vi "ql2_id_to_query.vi"(11 "id":u32) -> (3 "query_type":T1)   [LabVIEW 2017, in "rethinkdb.lvlib"]
uses:
  ql2_query.ctl
  rethinkdb.lvlib
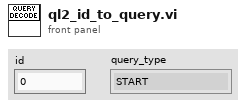
[diagram p1: front panel]
types:
  T1 = typedef "rethinkdb.lvlib/ql2_query.ctl" = enum8{"START", "CONTINUE", "STOP", "NOREPLY_WAIT", "SERVER_INFO", "invalid"}
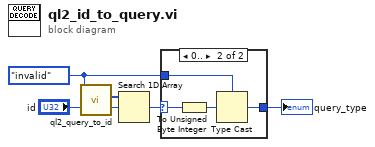
[diagram p0: block diagram]
diagram:
  w1 = ql2_query."invalid" ("query_type")
  n1 = call "ql2_query_to_id.vi"("query_type"=w1) -> ("query_type_ids"=w2:u32[])  [unwired: 9 in, 1 out]
  n2 = Search 1D Array(1D array=w2, element="id") -> (index of element=w4:i32)  [unwired: 1 in]
  n3 = case shown="0.." w4 {
    selector: w4 -> [_ w7]
    tunnel: [w6 w10] -> w3
    tunnel: w1 -> [w6 w9]
    frame ..-1 {
    }
    frame 0.. {
      n4 = To Unsigned Byte Integer(number=w7) -> (unsigned 8bit integer=w8:u8)
      n5 = Type Cast(type=w9, x=w8) -> (*(type *) &x=w10:T1)
    }
  }
  "query_type" <- w3
